vi "Get BER Floor.vi"(8 "error in":errorcluster, 11 "eye scan in":refnum<class "niHighSpeedSerial Eye Scan v1 Host.lvclass">) -> (0 "error out":errorcluster, 2 "BER floor":dbl, 3 "eye scan out":refnum<class "niHighSpeedSerial Eye Scan v1 Host.lvclass">)   [LabVIEW 2015, in "niHighSpeedSerial Eye Scan v1 Host.lvclass"]
doc: "Returns the coerced <b>BER (Bit Error Rate) Floor</b>. Note that the returned value is computed based off of the prescale and may be smaller than what was requested.\n\n<B>Input Parameters</B>\n\n<B>error in</B> describes error conditions that occur before this node runs. This input provides standard 'error in' functionality.\n\n<B>eye scan in</B> Takes in a reference to your session from the previous VI.\n\n<B>Output Parameters</B>\n\n<B>error out</B> contains error information. This output provides standard 'error out' functionality.\n\n<B>eye scan out</B> passes a reference to your session to the next VI.\n\n<B>BER floor</B> is the minimum Bit Error Rate which may be computed."
uses:
  <instrlib>/niHighSpeedSerial/Eye Scan/v1/Host/Eye Scan/niHighSpeedSerial Eye Scan v1 Host.lvclass
  <instrlib>/niHighSpeedSerial/Eye Scan/v1/Host/Eye Scan/niHighSpeedSerial Eye Scan v1 Host.lvclass/niHighSpeedSerial Eye Scan v1 Host.ctl
  <instrlib>/niHighSpeedSerial/Eye Scan/v1/Host/Common/Public/Equalization Mode.ctl
  <instrlib>/niHighSpeedSerial/Eye Scan/v1/Host/Common/niHighSpeedSerial Eye Scan Common v1 Host.lvlib
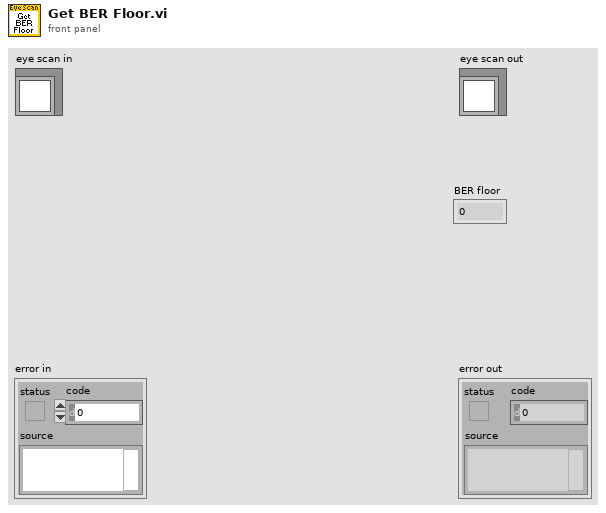
[diagram p1: front panel]
types:
  T1 = typedef "niHighSpeedSerial Eye Scan Common v1 Host.lvlib/Equalization Mode.ctl" = enum16{"DFE", "LPM"}
  T2 = typedef "niHighSpeedSerial Eye Scan v1 Host.lvclass/Private Data.ctl" = cluster{"instruction target":refnum<class "niInstr Instruction Target v1 Host.lvclass">, "channels":T3[], "measure state":T4, "rx output divider":T5, "equalization mode":T1, "rx internal data width":T6, "BER floor":dbl, "number of points completed":i32, "rx output divider configured?":bool, "equalization mode configured?":bool, "rx data width configured?":bool}
  T3 = typedef "niHighSpeedSerial Eye Scan v1 Host.lvclass/Channel Data.ctl" = cluster{"instance":u8, "channel":refnum<class "niHighSpeedSerial Eye Scan Single Point v1 Host.lvclass">, "point iterator":refnum<class "niHighSpeedSerial Eye Scan Point Iterator v1 Host.lvclass">}
  T4 = typedef "niHighSpeedSerial Eye Scan v1 Host.lvclass/Measure State.ctl" = enum16{"Uninitialized", "Initialized", "Ready", "Measuring", "Finished", "Aborted"}
  T5 = typedef "niHighSpeedSerial Eye Scan Common v1 Host.lvlib/RX Output Divider.ctl" = enum16{"1", "2", "4", "8", "16"}
  T6 = typedef "niHighSpeedSerial Eye Scan Common v1 Host.lvlib/Data Width.ctl" = enum16{"16 Bit", "20 Bit", "32 Bit", "40 Bit"}
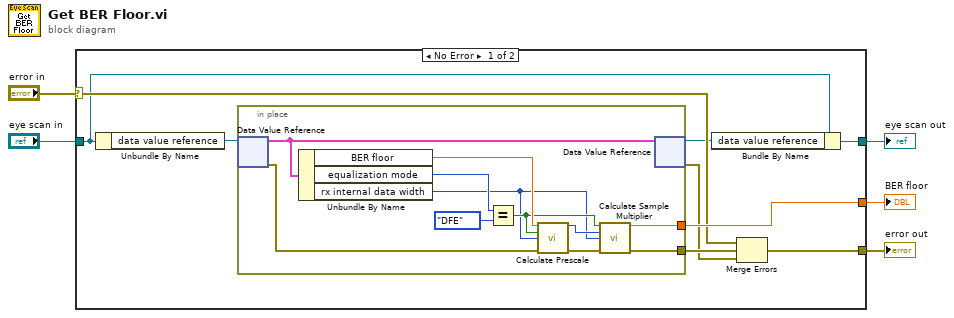
[diagram p0: block diagram]
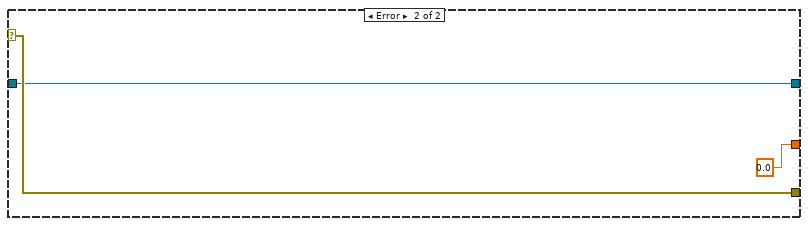
[diagram p2: hidden frame]
diagram:
  n1 = case shown="No Error" "error in" {
    selector: "error in" -> [w10 w28]
    tunnel: [w9 w28] -> w4
    tunnel: [w6 w27] -> w2
    tunnel: "eye scan in" -> [w7 w27]
    tunnel: [w13 0.0 ("BER Floor")] -> w1
    frame No Error {
      n2 = Unbundle By Name(w7) -> ("data value reference"=w14:refnum<data-value>)
      n3 = in-place {
        in-place-border: [w16] -> w13
        in-place-border: [w19] -> w12
        n4 = in-place-dvr #1(w14) -> (w25:T2, w21:errorcluster)
        n5 = Unbundle By Name(w25) -> ("BER floor"=w24:dbl, "equalization mode"=w23:T1, "rx internal data width"=w15:T6)
        n6 = Equal?(x=w23, y=Equalization_Mode."DFE" ("Equalization Mode")) -> (x = y?=w17:bool)
        n7 = call <instrlib>:"Calculate Prescale.vi"("minimum BER"=w24, "in DFE mode?"=w17, "receiver data width"=w15, "error in"=w21) -> ("prescale"=w18:u8, "error out"=w20:errorcluster)  [unwired: 10 in]
        n8 = call <instrlib>:"Calculate Sample Multiplier.vi"("in DFE mode?"=w17, "prescale"=w18, "receiver data width"=w15, "error in"=w20) -> ("BER floor"=w16:dbl, "error out"=w19:errorcluster)  [unwired: 9 in, 1 out]
        n9 = in-place-dvr #1(w25) -> (w8:refnum<data-value>, w11:errorcluster)
      }
      n10 = Bundle By Name(cluster=w7, "data value reference"=w8) -> (w6:refnum<class "niHighSpeedSerial Eye Scan v1 Host.lvclass">)
      n11 = Merge Errors(w10, w12, w11) -> (w9:errorcluster)
    }
    frame Error {
    }
  }
  "error out" <- w4
  "eye scan out" <- w2
  "BER floor" <- w1
